vi "Get INI Data.vi"(8 "error in":errorcluster, 11 "Section":string="Setting") -> (0 "error out":errorcluster, 3 "INI Data":T1(array[cluster]))   [LabVIEW 2019]
uses:
  Controls/KeyValue.ctl
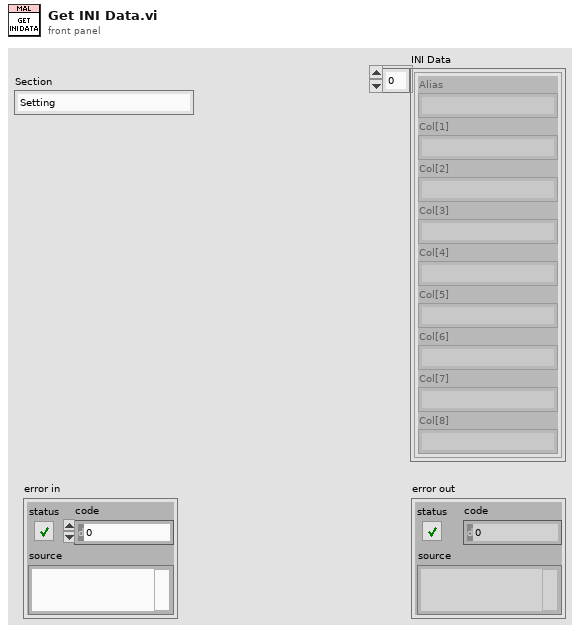
[diagram p1: front panel]
types:
  T1 = cluster{"Alias":string, "Col[1]":string, "Col[2]":string, "Col[3]":string, "Col[4]":string, "Col[5]":string, "Col[6]":string, "Col[7]":string, "Col[8]":string}[]
  T2 = typedef "KeyValue.ctl" = cluster{"Key":string, "Value":string}
  T3 = typedef "MAL.lvlib/INI DataType.ctl" = cluster{"Section":string, "Data":variant}
  T4 = cluster{"string array[0]":string, "string array[1]":string, "string array[2]":string, "string array[3]":string, "string array[4]":string, "string array[5]":string, "string array[6]":string, "string array[7]":string, "string array[8]":string}
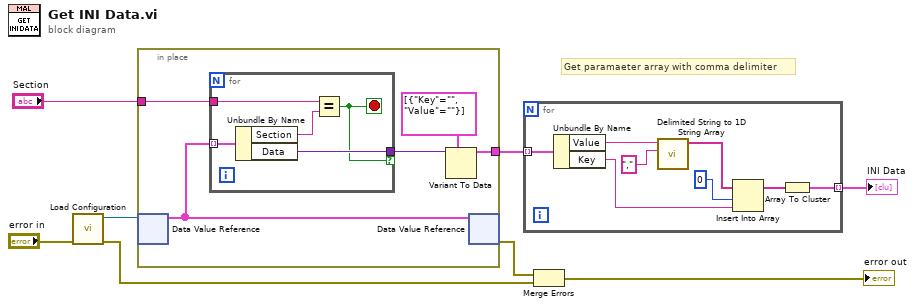
[diagram p0: block diagram]
diagram:
  # "Get paramaeter array with comma delimiter"
  n1 = call "Load Configuration.vi"("error in"="error in") -> ("error out"=w8:errorcluster, "Config DVR"=w6:refnum<data-value>)  [unwired: 9 in]
  n2 = in-place {
    in-place-border: [w11] -> w5
    in-place-border: "Section" -> [w9]
    n3 = in-place-dvr #1(w6) -> (w12:T3[])  [unwired: 1 out]
    n4 = for {
      tunnel: w12 -> [w18] mode=indexing
      tunnel: [w16] -> w13 if=w15
      tunnel: w9 -> [w14]
      stop <- w15 stop-if-true
      n5 = Unbundle By Name(w18) -> ("Section"=w17:string, "Data"=w16:variant)
      n6 = Equal?(x=w14, y=w17) -> (x = y?=w15:bool)
    }
    n7 = Variant To Data(type=T2[] [{"Key"="", "Value"=""}], Variant=w13) -> (data=w11:T2[])  [unwired: 1 in, 1 out]
    n8 = in-place-dvr #1(w12) -> (w7:errorcluster)  [unwired: 1 out]
  }
  n9 = for {
    tunnel: w5 -> [w25] mode=indexing
    tunnel: [w19] -> w1 mode=indexing
    n10 = Unbundle By Name(w25) -> ("Value"=w24:string, "Key"=w22:string)
    n11 = call <vilib>:"Delimited String to 1D String Array.vi"("delimiter"=",", "delimited string"=w24) -> ("string array"=w23:string[])  [unwired: 9 in]
    n12 = Insert Into Array(array=w23, index=0, new element=w22) -> (w20:string[])
    n13 = Array To Cluster(array=w20) -> (cluster=w19:T4)
  }
  "INI Data" <- w1
  n14 = Merge Errors(w7, w8) -> (→"error out":errorcluster)
